vi "Get Execution Units.vi"(8 "error in":errorcluster, 11 "custom device ref":T1 format="%.0x") -> (0 "error out":errorcluster, 1 "List of Execution Units":string[](array[string]), 2 "Execution Units Refs":T1[](array[typedef]) format="%.0x", 3 "custom device ref out":T1 format="%.0x")   [LabVIEW 2020, in "AIM ARINC 664 Scripting.lvlib"]
uses:
  AIM ARINC 664 Scripting.lvlib
  <vilib>/NI VeriStand/Custom Device API/Custom Device Item Ref.ctl
  <vilib>/NI VeriStand/Custom Device API/Custom Device API.lvlib
  <vilib>/Utility/SystemLogging/NI_SystemLogging.lvlib
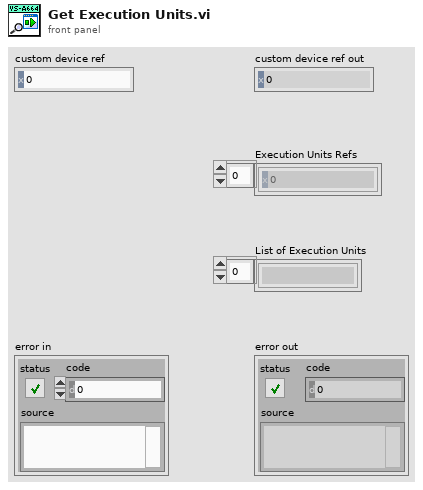
[diagram p1: front panel]
types:
  T1 = typedef "Custom Device API.lvlib/Custom Device Item Ref.ctl" = u64
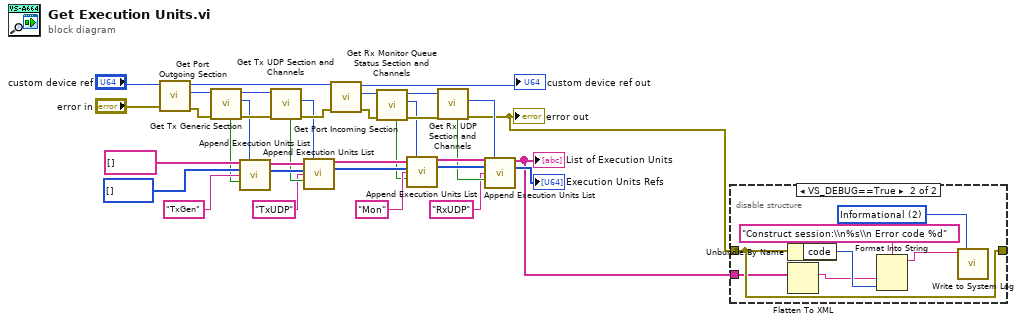
[diagram p0: block diagram]
diagram:
  n1 = call "Get Port Outgoing Section.vi"("error in"="error in", "Port Ref"="custom device ref") -> ("error out"=w33:errorcluster, "Outgoing Section Ptr"=w34:T1, "Port Ref out"=w32:T1)  [unwired: 6 in, 1 out]
  n2 = call "Get Tx Generic Section.vi"("error in"=w33, "Parent section Ref in"=w34) -> ("error out"=w22:errorcluster, "Item Ref"=w19:T1, "Parent section Ref out"=w21:T1, "Found?"=w20:bool)  [unwired: 6 in]
  n3 = call "Append Execution Units List.vi"("Input List"=string[] [] ("appended array"), "Item Ref"=w19, "Input Refs"=T1[] [] ("appended array"), "Execution Unit Name"="TxGen", "Found?"=w20) -> ("List Out"=w27:string[], "Ref Out"=w26:T1[])  [unwired: 9 in]
  n4 = call "Get Tx UDP Section and Channels.vi"("error in"=w22, "Custom Device Ref in"=w21) -> ("error out"=w16:errorcluster, "Section Ref out"=w3:T1, "Found?"=w18:bool)  [unwired: 5 in, 2 out]
  n5 = call "Append Execution Units List.vi"("Input List"=w27, "Item Ref"=w3, "Input Refs"=w26, "Execution Unit Name"="TxUDP", "Found?"=w18) -> ("List Out"=w15:string[], "Ref Out"=w13:T1[])  [unwired: 9 in]
  n6 = call "Get Port Incoming Section.vi"("error in"=w16, "Port Ref"=w32) -> ("error out"=w25:errorcluster, "Incoming Ref out"=w24:T1, "Port Ref out"=→"custom device ref out":T1)  [unwired: 6 in, 1 out]
  n7 = call "Get Rx Monitor Queue Status Section and Channels.vi"("error in"=w25, "Custom Device Ref in"=w24) -> ("error out"=w10:errorcluster, "Monitor Queue Status Section Ref out"=w9:T1, "Custom Device Ref out"=w23:T1, "Found?"=w6:bool)  [unwired: 5 in, 1 out]
  n8 = call "Append Execution Units List.vi"("Input List"=w15, "Item Ref"=w9, "Input Refs"=w13, "Execution Unit Name"="Mon", "Found?"=w6) -> ("List Out"=w14:string[], "Ref Out"=w12:T1[])  [unwired: 9 in]
  n9 = call "Get Rx UDP Section and Channels.vi"("error in"=w10, "Custom Device Ref in"=w23) -> ("error out"=w2:errorcluster, "Tx Queue Status Section Ref out"=w8:T1, "Found?"=w5:bool)  [unwired: 5 in, 2 out]
  "error out" <- w2
  n10 = call "Append Execution Units List.vi"("Input List"=w14, "Item Ref"=w8, "Input Refs"=w12, "Execution Unit Name"="RxUDP", "Found?"=w5) -> ("List Out"=w1:string[], "Ref Out"=→"Execution Units Refs":T1[])  [unwired: 9 in]
  "List of Execution Units" <- w1
  n11 = disable-structure shown="VS_DEBUG==True" {
    disable-tunnel: w2 -> [_ w39]
    disable-tunnel: [_ w39] -> _
    disable-tunnel: w1 -> [_ w38]
    frame condition #0 {
    }
    frame condition #1 (active) {
      w41 = 2 items=["Error", "Warning", "Informational"] ("severity")
      n12 = Unbundle By Name(w39) -> ("code"=w40:i32)
      n13 = Flatten To XML(6:w38) -> (2:w37:string)
      n14 = Format Into String(format string="Construct session:\\n%s\\n Error code %d", w37, w40) -> (resulting string=w42:string)  [unwired: 2 in, 1 out]
      n15 = call <vilib>:"Write to System Log.vi"("severity"=w41, "message"=w42) -> ()  [unwired: 9 in, 1 out]
    }
  }
